vi "IMU read.vi"(11 "error in (no error)":errorcluster) -> (0 "Gyro deg/s":cluster{dbl, dbl, dbl}, 1 "Frames Read":u16[](array[numeric]), 2 "Accel, Gyro":u16[](array[numeric]), 3 "error out":errorcluster, 4 "Accel g's":cluster{dbl, dbl, dbl}, 6 "Accel g's 2":dbl[](array[numeric]), 8 "Gyro deg/s 2":dbl[](array[numeric]))   [LabVIEW 2016]
uses:
  <vilib>/myRIO/Instrument Drivers/Onboard IO/DIO/typedefs/DIO Reference.ctl
  <vilib>/myRIO/Common/Instrument Driver Framework/Utilities/typedefs/myRIO Generic Hardware Reference.ctl
  <vilib>/myRIO/Common/Instrument Driver Framework/Utilities/typedefs/Hardware Version Enum.ctl
  <vilib>/myRIO/Common/Instrument Driver Framework/Utilities/typedefs/myRIO v1.0 Reference.ctl
  <vilib>/myRIO/Common/Instrument Driver Framework/Utilities/typedefs/Generic FPGA Reference.ctl
  <vilib>/myRIO/Common/Instrument Driver Framework/myRIO v1.0/DIO/typedefs/DIO Channels List.ctl
  <vilib>/myRIO/Common/Instrument Driver Framework/myRIO v1.0/DIO/typedefs/DIO Channels Enum.ctl
  <vilib>/userdefined/High Color/nirio_resource_hc.ctl
  <vilib>/myRIO/Instrument Drivers/Onboard IO/SPI/typedefs/SPI User Configuration.ctl
  <vilib>/myRIO/Common/Instrument Driver Framework/myRIO v1.0/SPI/typedefs/SPI Clock Phase.ctl
  <vilib>/myRIO/Common/Instrument Driver Framework/myRIO v1.0/SPI/typedefs/SPI Clock Polarity.ctl
  <vilib>/myRIO/Common/Instrument Driver Framework/myRIO v1.0/SPI/typedefs/SPI Data Direction.ctl
  <vilib>/myRIO/Common/Instrument Driver Framework/myRIO v1.0/SPI/typedefs/SPI Frame Length.ctl
  <vilib>/myRIO/Instrument Drivers/Onboard IO/SPI/typedefs/SPI Reference.ctl
  <vilib>/myRIO/Common/Instrument Driver Framework/myRIO v1.0/SPI/typedefs/SPI Channels Enum.ctl
  <vilib>/myRIO/Instrument Drivers/Onboard IO/SPI/typedefs/SPI Configuration.ctl
  <vilib>/myRIO/Common/Instrument Driver Framework/Utilities/vis/Is FPGA Ref Available.vi
  <vilib>/myRIO/Common/Instrument Driver Framework/roboRIO v1.0/DIO/vis/roboRIO v1.0 Open DIO.vi
  <vilib>/myRIO/Instrument Drivers/Onboard IO/DIO/vis/Write.vi
  <vilib>/myRIO/Common/Instrument Driver Framework/roboRIO v1.0/SPI/vis/roboRIO v1.0 Open SPI.vi
  <vilib>/myRIO/Instrument Drivers/Onboard IO/SPI/vis/Configure.vi
  <vilib>/myRIO/Instrument Drivers/Onboard IO/SPI/vis/Write Read.vi
  <vilib>/myRIO/Common/Instrument Driver Framework/Utilities/vis/Validate Channels.vi
  <vilib>/myRIO/Common/Instrument Driver Framework/roboRIO v1.0/DIO/vis/roboRIO v1.0 Reserve DIO.vi
  <vilib>/myRIO/Common/Instrument Driver Framework/roboRIO v1.0/SPI/vis/roboRIO v1.0 Reserve SPI.vi
  <vilib>/myRIO/Common/Instrument Driver Framework/roboRIO v1.0/DIO/vis/roboRIO v1.0 Build MUX Configuration DIO.vi
  <vilib>/myRIO/Common/Instrument Driver Framework/roboRIO v1.0/Resource Manager/vis/roboRIO v1.0 Reserve Channel List.vi
  <vilib>/myRIO/Common/Instrument Driver Framework/roboRIO v1.0/SPI/vis/roboRIO v1.0 Build MUX Configuration SPI.vi
  <vilib>/myRIO/Common/Instrument Driver Framework/roboRIO v1.0/Resource Manager/vis/roboRIO v1.0 Create Configuration List.vi
  <vilib>/myRIO/Common/Instrument Driver Framework/roboRIO v1.0/Resource Manager/vis/roboRIO v1.0 Reserve Channel.vi
  <vilib>/myRIO/Common/Instrument Driver Framework/roboRIO v1.0/Resource Manager/vis/roboRIO v1.0 Unreserve Channel.vi
  <vilib>/myRIO/Common/Instrument Driver Framework/myRIO v1.0/Resource Manager/vis/myRIO v1.0 Create Configuration List.vi
  <vilib>/myRIO/Common/Instrument Driver Framework/roboRIO v1.0/Resource Manager/vis/roboRIO v1.0 Build Mutex Name.vi
  <vilib>/Utility/VariantDataType/GetNumericInfo.vi
  <vilib>/Utility/error.llb/Error Cluster From Error Code.vi
  <vilib>/myRIO/Common/Instrument Driver Framework/roboRIO v1.0/roboRIO v1.0 Open.vi
  <vilib>/myRIO/Common/Instrument Driver Framework/Utilities/vis/IO Manager.vi
  <vilib>/myRIO/Common/Instrument Driver Framework/Utilities/vis/Configuration Manager.vi
  <vilib>/myRIO/Common/Instrument Driver Framework/roboRIO v1.0/Resource Manager/vis/roboRIO v1.0 Configure IO.vi
  <vilib>/myRIO/Common/Instrument Driver Framework/myRIO v1.0/myRIO v1.0 Close.vi
  <vilib>/myRIO/Common/Instrument Driver Framework/roboRIO v1.0/DIO/vis/roboRIO v1.0 Write DIO.vi
  <vilib>/myRIO/Common/Instrument Driver Framework/roboRIO v1.0/SPI/vis/roboRIO v1.0 Configure SPI.vi
  <vilib>/myRIO/Common/Instrument Driver Framework/roboRIO v1.0/SPI/vis/roboRIO v1.0 Write Read SPI.vi
  <vilib>/myRIO/Express VI/Onboard IO/DO/DO Express VI.xnode
  <vilib>/myRIO/Instrument Drivers/Onboard IO/DIO/vis/myRIO DIO Open.xnode
  <vilib>/myRIO/Express VI/Onboard IO/SPI/SPI Express VI.xnode
  <vilib>/myRIO/Instrument Drivers/Onboard IO/SPI/vis/myRIO SPI Open.xnode
  <vilib>/myRIO/Instrument Drivers/Onboard IO/DIO/DIO.lvlib
  <vilib>/myRIO/Instrument Drivers/Onboard IO/SPI/SPI.lvlib
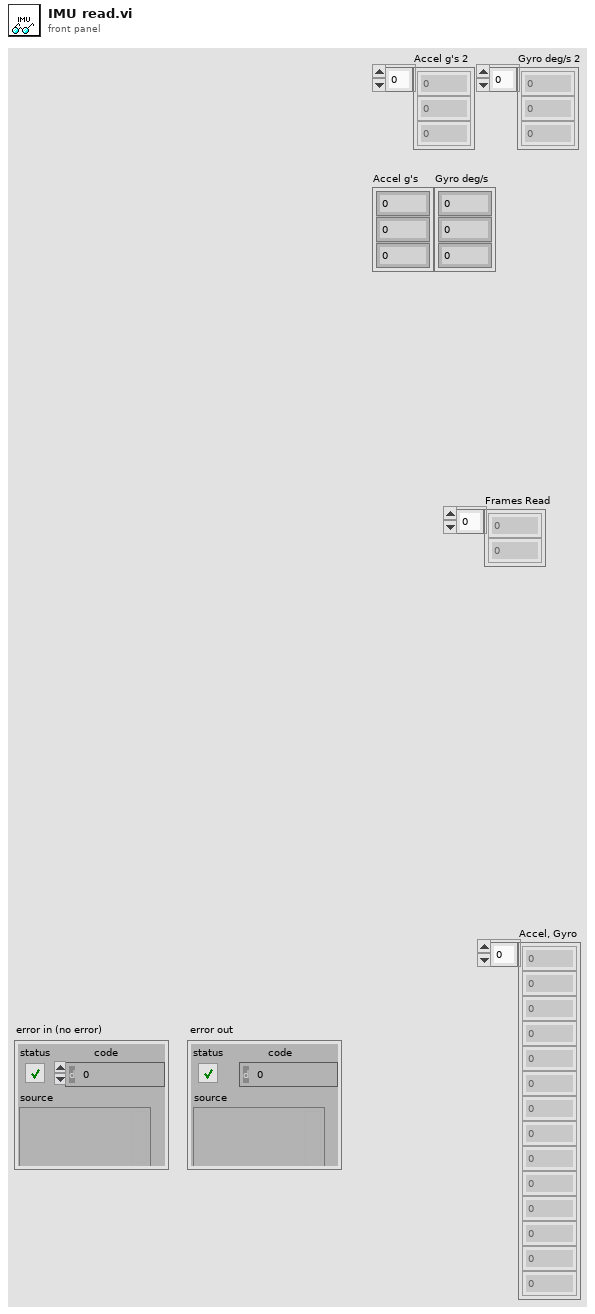
[diagram p1: front panel]
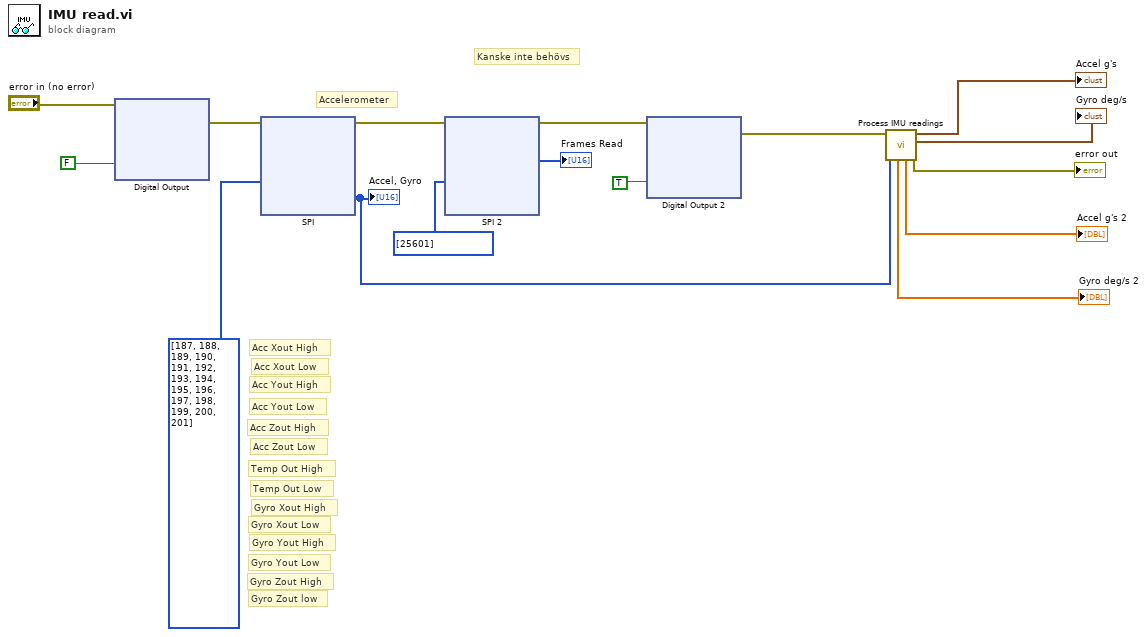
[diagram p0: block diagram]
diagram:
  # "Kanske inte behövs"
  # "Gyro Zout low"
  # "Gyro Zout High"
  # "Gyro Yout Low"
  # "Gyro Yout High"
  # "Gyro Xout Low"
  # "Gyro Xout High"
  # "Temp Out Low"
  # "Temp Out High"
  # "Acc Zout Low"
  # "Acc Zout High"
  # "Acc Yout Low"
  # "Acc Yout High"
  # "Acc Xout Low"
  # "Acc Xout High"
  # "Accelerometer"
  n1 = xnode "Digital Output"("SPI/CS0 (Pin 2)"=FALSE ("Chip Select (A/DIO0 (Pin 11))"), "error in (no error)"="error in (no error)") -> ("error out"=w14:errorcluster)
  n2 = xnode "SPI"("Frames to Write"=u16[] [187, 188, 189, 190, 191, 192, 193, 194, 195, 196, 197, 198, 199, 200, 201], "error in (no error)"=w14) -> ("Frames Read"=w6:u16[], "error out"=w8:errorcluster)
  "Accel, Gyro" <- w6
  n3 = xnode "SPI 2"("Frames to Write"=u16[] [25601], "error in (no error)"=w8) -> ("Frames Read"=→"Frames Read":u16[], "error out"=w7:errorcluster)
  n4 = xnode "Digital Output 2"("SPI/CS0 (Pin 2)"=TRUE ("Chip Select (A/DIO0 (Pin 11))"), "error in (no error)"=w7) -> ("error out"=w5:errorcluster)
  n5 = call "Process IMU readings.vi"("Sensor Data in"=w6, "error in (no error)"=w5) -> ("error out"=→"error out":errorcluster, 2:"Gyro deg/s"=→"Gyro deg/s":cluster{dbl, dbl, dbl}, 3:"Accel g's"=→"Accel g's":cluster{dbl, dbl, dbl}, 4:"Accel g's"=→"Accel g's 2":dbl[], 6:"Gyro deg/s"=→"Gyro deg/s 2":dbl[])  [unwired: 5 in]
